vi "subSplitProjectForTargetTypes.vi"(8 "error in (no error)":errorcluster, 11 "SolutionBuilder in":refnum<class "SolutionBuilder.lvclass">) -> (0 "error out":errorcluster, 3 "SolutionBuilder out":refnum<class "SolutionBuilder.lvclass">)   [LabVIEW 2019, in "SolutionBuilder.lvlib" / "SolutionBuilder.lvclass"]
uses:
  SolutionBuilder.lvclass
  SolutionBuilder.lvclass/SolutionBuilder.ctl
  <vilib>/xml/Load XML File.vi
  <vilib>/xml/Close Reference(Node).vi
  <vilib>/xml/NI_XML.lvlib
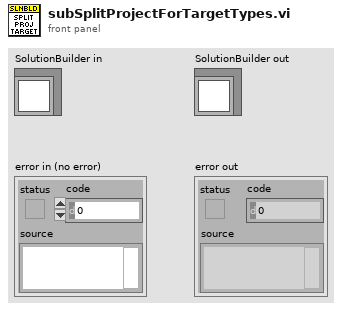
[diagram p1: front panel]
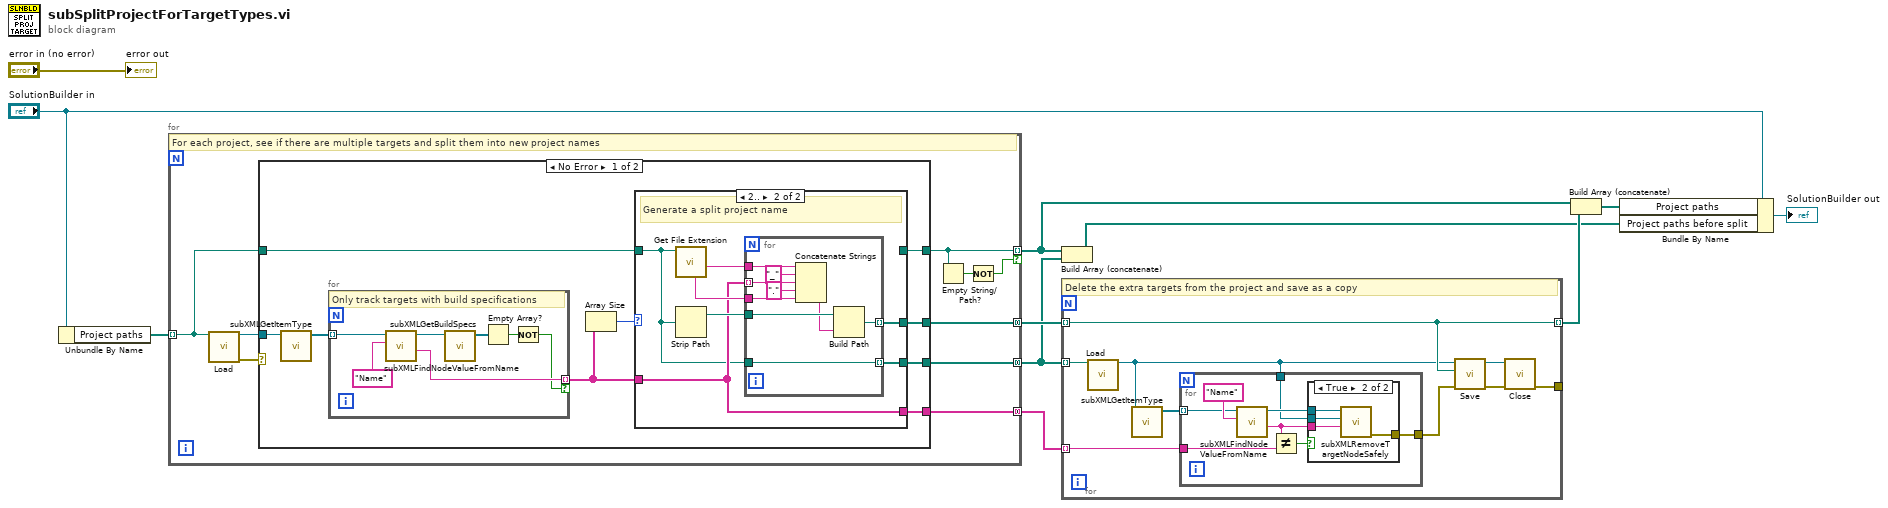
[diagram p0: block diagram]
diagram:
  n1 = Unbundle By Name("SolutionBuilder in") -> ("Project paths"=w10:path[])
  n2 = for {
    tunnel: w10 -> [w18] mode=indexing
    tunnel: [w17] -> w9 mode=concatenating
    tunnel: [w16] -> w8 mode=concatenating
    tunnel: [w15] -> w2 mode=concatenating
    tunnel: [w14] -> w3 mode=indexing if=w12
    # "For each project, see if there are multiple targets and split them into new project names"
    n3 = call-poly <vilib>:"Load.vi"("path to XML document"=w18) -> ("DOM document out"=w19:refnum<k20>, "error out"=w20:errorcluster)  [unwired: 12 in, 1 out]
    n4 = case shown="No Error" w20 {
      tunnel: w19 -> [w26 _]
      tunnel: w18 -> [w25 w54]
      tunnel: [w24 _] -> w17
      tunnel: [w23 _] -> w16
      tunnel: [w22 _] -> w15
      tunnel: [w21 w54] -> w14
      frame No Error {
        n5 = call "subXMLGetItemType.vi"("Refnum in"=w26) -> ("Nodes"=w29:refnum<k20>[])  [unwired: 10 in]
        n6 = for {
          tunnel: w29 -> [w52] mode=indexing
          tunnel: [w51] -> w27 mode=indexing if=w47
          # "Only track targets with build specifications"
          n7 = call "subXMLFindNodeValueFromName.vi"("Property name"="Name", "Refnum in"=w52) -> ("Value"=w51:string, "Refnum out"=w50:refnum<k20>)  [unwired: 7 in, 1 out]
          n8 = call "subXMLGetBuildSpecs.vi"("Refnum in"=w50) -> ("Nodes"=w49:refnum<k20>[])  [unwired: 9 in, 1 out]
          n9 = Empty Array?(array=w49) -> (empty?=w48:bool)
          n10 = Not(x=w48) -> (.not. x?=w47:bool)
        }
        n11 = Array Size(array=w27) -> (size(s)=w28:i32)
        n12 = case shown="2.." w28 {
          tunnel: w27 -> [_ w33]
          tunnel: w25 -> [w30 w31]
          tunnel: [_ w34] -> w24
          tunnel: [_ w33] -> w23
          tunnel: [_ w32] -> w22
          tunnel: [w30 _] -> w21
          frame Default {
            # "Keep the existing project the same"
          }
          frame 2.. {
            # "Generate a split project name"
            n13 = call <vilib>:"Get File Extension.vi"("file"=w31) -> ("filename without extension"=w36:string, "unmodified file extension"=w37:string)  [unwired: 6 in, 3 out]
            n14 = Strip Path(path=w31) -> (stripped path=w35:path)  [unwired: 1 out]
            n15 = for {
              tunnel: w37 -> [w44]
              tunnel: w36 -> [w46]
              tunnel: w35 -> [w42]
              tunnel: w33 -> [w43] mode=indexing
              tunnel: [w40] -> w34 mode=indexing
              tunnel: [w39] -> w32 mode=indexing
              tunnel: w31 -> [w39]
              n16 = Concatenate Strings(w46, "_" ("string"), w43, "." ("string"), w44) -> (w41:string)
              n17 = Build Path(base path=w42, name or relative path=w41) -> (appended path=w40:path)
            }
          }
        }
      }
      frame Error {
      }
    }
    n18 = Empty String/Path?(string/path=w14) -> (empty?=w13:bool)
    n19 = Not(x=w13) -> (.not. x?=w12:bool)
  }
  n20 = Build Array (concatenate)(w3, w2) -> (w1:path[])
  n21 = for {
    tunnel: w2 -> [w62] mode=indexing
    tunnel: w9 -> [w56] mode=indexing
    tunnel: w8 -> [w61] mode=indexing
    tunnel: [w57] -> _
    tunnel: [w56] -> w7 mode=indexing
    # "Delete the extra targets from the project and save as a copy"
    n22 = call-poly <vilib>:"Load.vi"("path to XML document"=w62) -> ("DOM document out"=w55:refnum<k20>)  [unwired: 12 in, 2 out]
    n23 = call "subXMLGetItemType.vi"("Refnum in"=w55) -> ("Nodes"=w63:refnum<k20>[])  [unwired: 10 in]
    n24 = for {
      tunnel: w63 -> [w70] mode=indexing
      tunnel: w61 -> [w67]
      tunnel: [w66] -> w58
      tunnel: w55 -> [w64]
      n25 = call "subXMLFindNodeValueFromName.vi"("Property name"="Name", "Refnum in"=w70) -> ("Value"=w65:string, "Refnum out"=w68:refnum<k20>)  [unwired: 7 in, 1 out]
      n26 = Not Equal?(x=w65, y=w67) -> (x != y?=w69:bool)
      n27 = case shown="True" w69 {
        tunnel: w68 -> [_ w74]
        tunnel: [_ w75] -> w66
        tunnel: w65 -> [_ w73]
        tunnel: w64 -> [_ w72]
        frame False {
        }
        frame True {
          n28 = call "subXMLRemoveTargetNodeSafely.vi"("Target name"=w73, "Document in"=w72, "Refnum in"=w74) -> ("error out"=w75:errorcluster)  [unwired: 8 in]
        }
      }
    }
    n29 = call <vilib>:"Save.vi"("error in (no error)"=w58, "XML file path"=w56, "DOM document in"=w55) -> ("error out"=w59:errorcluster, "DOM document out"=w60:refnum<k20>)  [unwired: 6 in, 1 out]
    n30 = call-poly <vilib>:"Close.vi"("error in (no error)"=w59, "node"=w60) -> ("error out"=w57:errorcluster)  [unwired: 7 in]
  }
  n31 = Build Array (concatenate)(w3, w7) -> (w5:path[])
  n32 = Bundle By Name(cluster="SolutionBuilder in", "Project paths"=w5, "Project paths before split"=w1) -> (→"SolutionBuilder out":refnum<class "SolutionBuilder.lvclass">)
  "error out" <- "error in (no error)"
